vi "APS set trigger manual.vi"(8 "error in (no error)":errorcluster caption="错误输入（无错误）", 10 "TrgCh":i32, 11 "Board_ID":i32) -> (0 "error out":errorcluster caption="错误输出", 3 "function return":i32)   [LabVIEW 2017, in "APS168.lvlib"]
doc: "I32 FNTYPE APS_set_trigger_manual( I32 Board_ID, I32 TrgCh );"
uses:
  APS168.lvlib
  APS168.dll
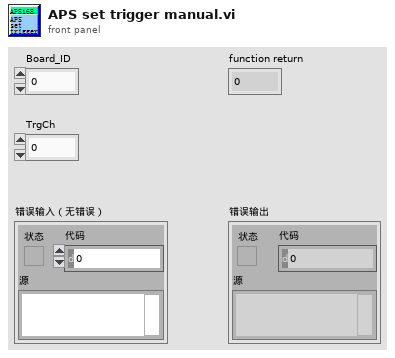
[diagram p1: front panel]
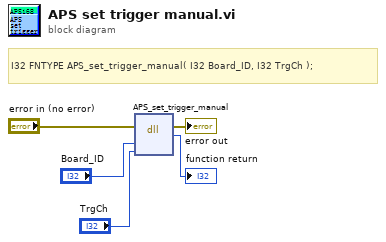
[diagram p0: block diagram]
diagram:
  # "I32 FNTYPE APS_set_trigger_manual( I32 Board_ID, I32 TrgCh );"
  n1 = dll-call lib="PTH2Gabs E迈治LV范例testSubVIsADLINKMotion204cAPS168.*" fn="APS_set_trigger_manual"(error in="error in (no error)", "Board_ID"="Board_ID", "TrgCh"="TrgCh") -> (error out=→"error out":errorcluster, →"function return":i32)  [unwired: 4 in, 1 out]
